vi "Read Allele-Bit.vi"(8 "error in (no error)":errorcluster, 11 "IGene in":refnum<class "IGene.lvclass">) -> (0 "error out":errorcluster, 2 "Allele-Bit":bool, 3 "IGene out":refnum<class "IGene.lvclass">)   [LabVIEW 2016, in "IGene.lvclass"]
uses:
  IGene.lvclass
  IGene.lvclass/IGene.ctl
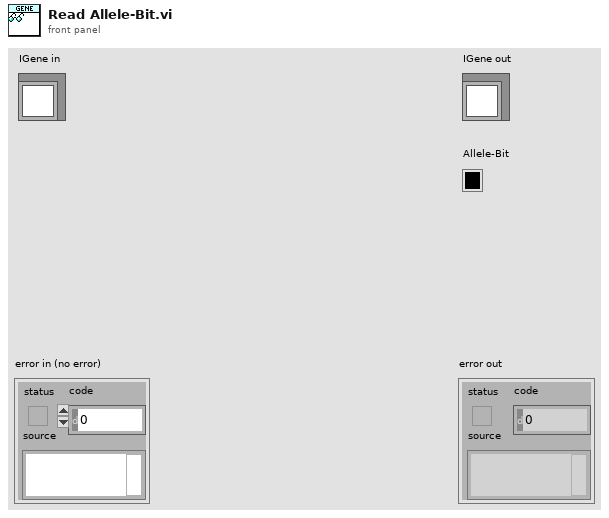
[diagram p1: front panel]
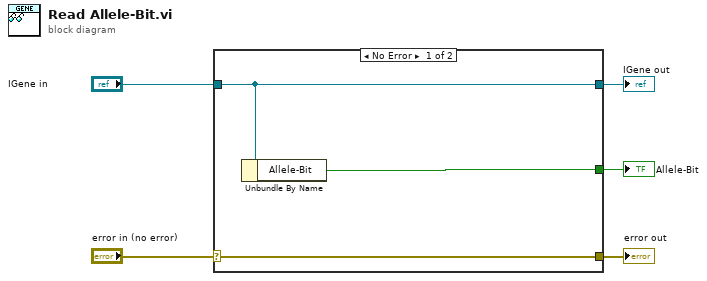
[diagram p0: block diagram]
diagram:
  n1 = case shown="No Error" "error in (no error)" {
    selector: "error in (no error)" -> [w8 w9]
    tunnel: [w8 w9] -> w4
    tunnel: [w7 w10] -> w2
    tunnel: "IGene in" -> [w7 w10]
    tunnel: [w6 _] -> w1
    frame No Error {
      n2 = Unbundle By Name(w7) -> ("Allele-Bit"=w6:bool)
    }
    frame Error {
    }
  }
  "error out" <- w4
  "IGene out" <- w2
  "Allele-Bit" <- w1
